vi "Find Line.vi"() -> ()   [LabVIEW 2016]
panel:
  out "return count":u32
  out "read buffer":string
  out "error out 2":errorcluster
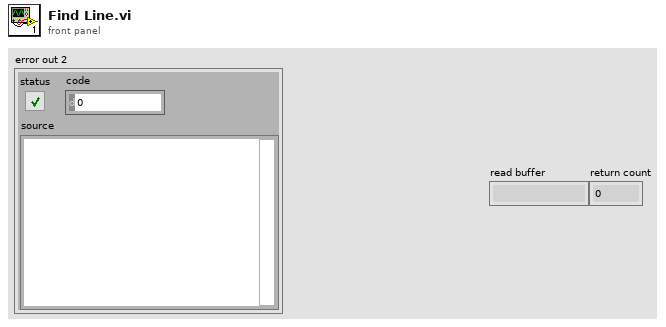
[diagram p1: front panel]
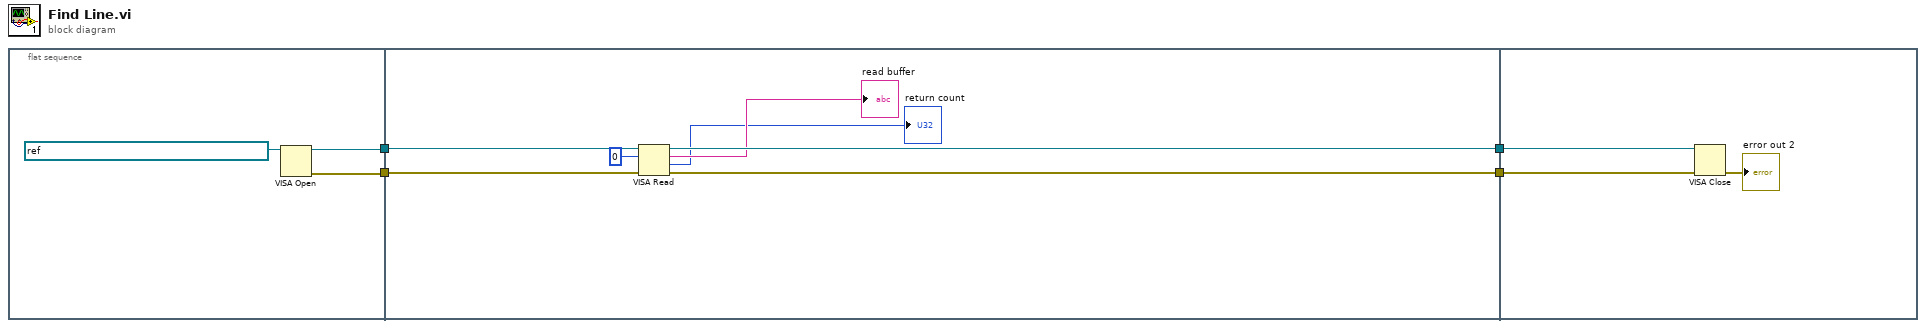
[diagram p0: block diagram]
diagram:
  n1 = flat-sequence {
    tunnel: [w7] -> w4
    tunnel: [w5] -> w2
    tunnel: w4 -> [w10]
    tunnel: [w14] -> w3
    tunnel: w2 -> [w9]
    tunnel: [w11] -> w1
    tunnel: w3 -> [w17]
    tunnel: w1 -> [w15]
    frame #0 {
      n2 = VISA Open(VISA resource name=refnum<visa-resource-name> "USB0::0xB1AC::0xF000::DEMO 0.0::0::RAW") -> (VISA resource name=w7:refnum<visa-resource-name>, error out=w5:errorcluster)  [unwired: 4 in]
    }
    frame #1 {
      n3 = VISA Read(VISA resource name=w10, byte count=u32 0, error in (no error)=w9) -> (VISA resource name out=w14:refnum<visa-resource-name>, read buffer=→"read buffer":string, return count=→"return count":u32, error out=w11:errorcluster)
    }
    frame #2 {
      n4 = VISA Close(VISA resource name=w17, error in (no error)=w15) -> (error out=→"error out 2":errorcluster)
    }
  }
